vi "SiosIfmSensorValue.vi"(1 "Sensor Number":i32, 2 "Device Number":i32) -> (0 "Requested Value":dbl)   [LabVIEW 2009]
uses:
  siosifm.dll
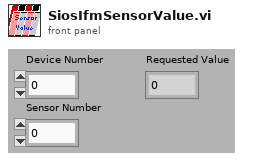
[diagram p1: front panel]
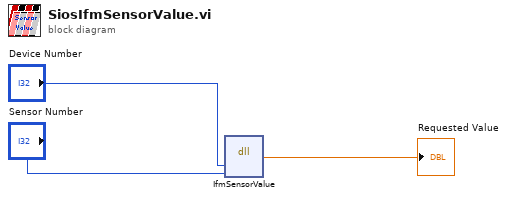
[diagram p0: block diagram]
diagram:
  n1 = dll-call lib="C:/WORK/Artem/RE-10/SIOS_IfmDLL/siosifm.dll" fn="IfmSensorValue"("devNumber"="Device Number", "sensor"="Sensor Number") -> ("requested_value"=→"Requested Value":dbl)  [unwired: 5 in, 2 out]
